vi "UpdateLinkCameraStatus.vi"(8 "error in (no error)":errorcluster, 10 "LinkCameraStatus":T1=enum."Connected", 11 "CameraTestingENI":refnum<class "CameraTestingENI.lvclass">) -> (0 "error out":errorcluster, 3 "CameraTestingENI":refnum<class "CameraTestingENI.lvclass">)   [LabVIEW 2020, in "CameraTestingProxy.lvlib" / "CameraTestingENI.lvclass"]
uses:
  CameraTestingENI.lvclass
  CameraTestingApp/ICameraTestingUI/TypeDef/LinkCameraStatus.ctl
  CameraTestingENI.lvclass/CameraTestingENI.ctl
  CameraTestingApp/ICameraTestingUI/TypeDef/ICameraTestingUI_typedef.lvlib
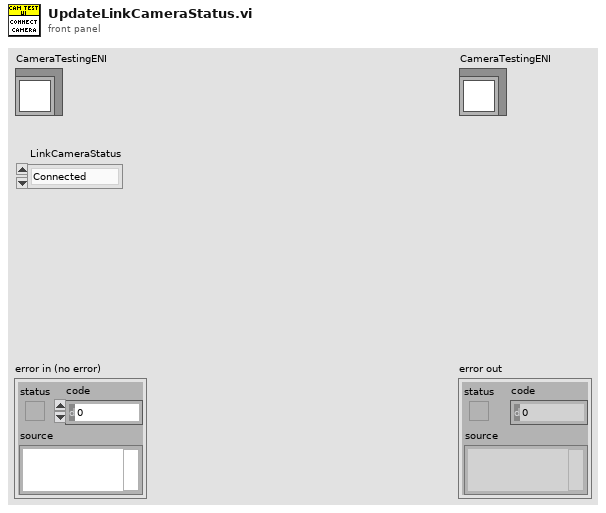
[diagram p1: front panel]
types:
  T1 = typedef "ICameraTestingUI_typedef.lvlib/LinkCameraStatus.ctl" = enum8{"Disconnected", "Connected", "Error"}
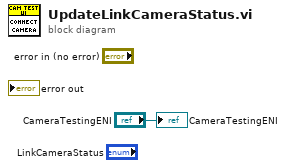
[diagram p0: block diagram]
diagram:
  "CameraTestingENI" <- "CameraTestingENI"
